vi "Get extended drive and motor status.vi"(0 "COM port":refnum<visa-resource-name>, 1 "Drive address":T5=1 items=["0", "1", "2", "3", "4", "5", "6", "7", "8", "9", "10", "11", "12", "13", "14", "15", "16", "17", "18", "19", "20", "21", "22", "23", "24", "25", "26", "27", "28", "29", "30", "31", "32", "33", "34", "35", "36", "37", "38", "39", "40", "41", "42", "43", "44", "45", "46", "47", "48", "49", "50", "51", "52", "53", "54", "55", "56", "57", "58", "59", "60", "61", "62", "63"]) -> (3 "No errors":bool, 4 "Modbus error cluster":T1={"Checksum ok"=FALSE, "Modbus exception code"=1, "Response from correct drive"=FALSE, "Comms error"={"status"=FALSE, "code"=0, "source"=""}} {"Modbus exception code" items=["None"=0, "Invalid function request"=1, "Invalid Modbus register address"=2, "Invalid / unauthorised data value"=3, "Device failure"=4, "Request accepted, wait"=5, "Drive busy"=6, "Request rejected"=7, "Memory parity error"=8, "Gateway path unavailable"=10, "Device failed to respond"=11]}, 5 "Extended drive status":T4, 6 "Motor data":T3)   [LabVIEW 2020]
doc: "Modbus RTU for Invertek drives. Paul Nathan 21-JUN-2022."
uses:
  ctls/Drive address.ctl
  ctls/Extended drive status bits.ctl
  ctls/Motor data.ctl
  ctls/Modbus error cluster.ctl
  ctls/Exception codes.ctl
  ctls/Register.ctl
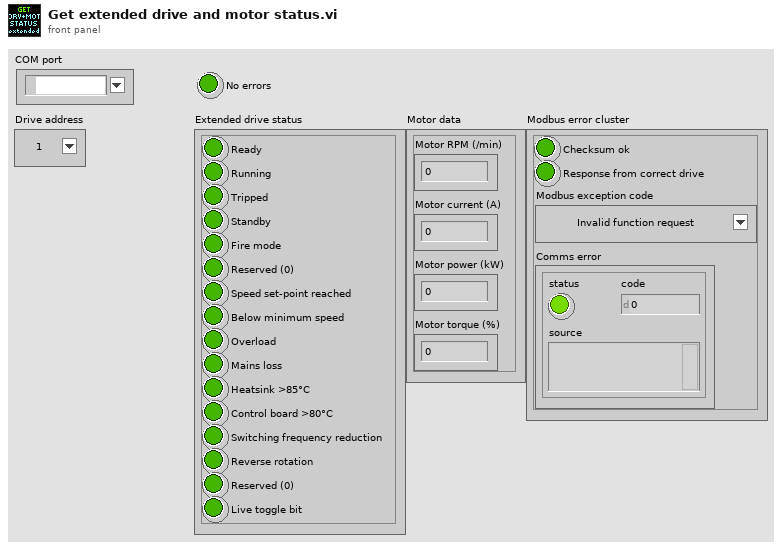
[diagram p1: front panel]
types:
  T1 = typedef "Modbus error cluster.ctl" = cluster{"Checksum ok":bool, "Modbus exception code":T2, "Response from correct drive":bool, "Comms error":errorcluster}
  T2 = typedef "Exception codes.ctl" = u8
  T3 = typedef "Motor data.ctl" = cluster{"Motor RPM (/min)":dbl, "Motor current (A)":dbl, "Motor power (kW)":dbl, "Motor torque (%)":dbl}
  T4 = typedef "Extended drive status bits.ctl" = cluster{"Ready":bool, "Running":bool, "Tripped":bool, "Standby":bool, "Fire mode":bool, "Reserved (0)":bool, "Speed set-point reached":bool, "Below minimum speed":bool, "Overload":bool, "Mains loss":bool, "Heatsink >85°C":bool, "Control board >80°C":bool, "Switching frequency reduction":bool, "Reverse rotation":bool, "Reserved (0)":bool, "Live toggle bit":bool}
  T5 = typedef "Drive address.ctl" = u8
  T6 = typedef "Register.ctl" = u16
  T7 = cluster{"Boolean array[0]":bool, "Boolean array[1]":bool, "Boolean array[2]":bool, "Boolean array[3]":bool, "Boolean array[4]":bool, "Boolean array[5]":bool, "Boolean array[6]":bool, "Boolean array[7]":bool, "Boolean array[8]":bool, "Boolean array[9]":bool, "Boolean array[10]":bool, "Boolean array[11]":bool, "Boolean array[12]":bool, "Boolean array[13]":bool, "Boolean array[14]":bool, "Boolean array[15]":bool}
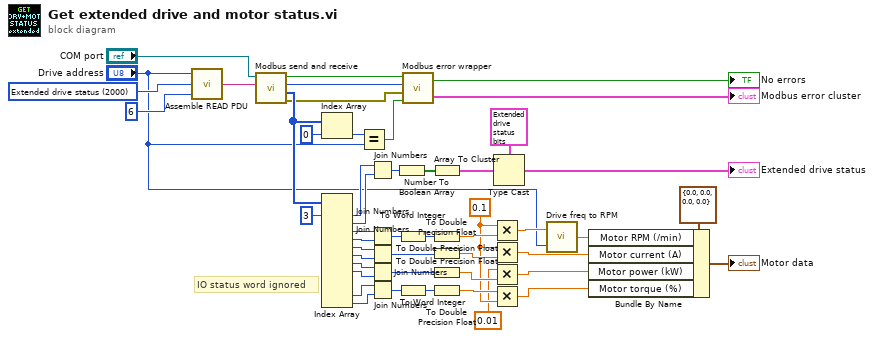
[diagram p0: block diagram]
diagram:
  w11 = T6 2000 items=["Control"=0, "RPM set-point"=4, "Drive status"=5, "Output RPM"=6, "Motor current"=7, "Motor torque"=8, "Motor power"=9, "DC bus voltage"=22, "Drive power stage temperature"=23, "kWh meter"=31, "MWh meter"=32, "Running time - hours"=33, "Running time - seconds"=34, "Internal drive temperature"=38, "Motor RMS voltage"=42, "Extended drive status"=2000] ("Register")
  w13 = 0.1 ("y")
  # "IO status word ignored"
  n1 = call "Assemble READ PDU.vi"("No. of registers"=u16 6, "Register"=w11, "Drive address"="Drive address") -> ("Ser out string"=w49:string)
  n2 = call "Modbus send and receive.vi"("Modbus telegram"=w49, "COM port"="COM port") -> ("Comms error"=w2:errorcluster, "Device response"=w44:u8[], "Modbus exception code"=w3:T2, "Checksum ok"=w4:bool)  [unwired: 2 in]
  n3 = Index Array(array=w44, index=0) -> (element=w46:u8)
  n4 = Index Array(array=w44, index #1=3 ("index")) -> (element #1=w38:u8, element #2=w37:u8, element #3=w24:u8, element #4=w23:u8, element #5=w22:u8, element #6=w21:u8, element #7=w20:u8, element #8=w19:u8, element #11=w18:u8, element #12=w17:u8)  [unwired: 11 in, 2 out]
  n5 = Equal?(x=w46, y="Drive address") -> (x = y?=w1:bool)
  n6 = Join Numbers(hi=w38, lo=w37) -> ((hi.lo)=w36:u16)
  n7 = Join Numbers(hi=w24, lo=w23) -> ((hi.lo)=w25:u16)
  n8 = Join Numbers(hi=w22, lo=w21) -> ((hi.lo)=w28:u16)
  n9 = Join Numbers(hi=w20, lo=w19) -> ((hi.lo)=w14:u16)
  n10 = Join Numbers(hi=w18, lo=w17) -> ((hi.lo)=w16:u16)
  n11 = Number To Boolean Array(number=w36) -> (Boolean array=w42:bool[])
  n12 = To Word Integer(number=w25) -> (16bit integer=w26:i16)
  n13 = To Word Integer(number=w16) -> (16bit integer=w15:i16)
  n14 = call "Modbus error wrapper.vi"("Response from correct drive"=w1, "Comms error"=w2, "Modbus exception code"=w3, "Checksum ok"=w4) -> ("Modbus error cluster"=→"Modbus error cluster":T1, "No errors"=→"No errors":bool)
  n15 = Array To Cluster(array=w42) -> (cluster=w41:T7)
  n16 = To Double Precision Float(number=w26) -> (double precision float=w29:dbl)
  n17 = To Double Precision Float(number=w28) -> (double precision float=w30:dbl)
  n18 = To Double Precision Float(number=w14) -> (double precision float=w31:dbl)
  n19 = To Double Precision Float(number=w15) -> (double precision float=w32:dbl)
  n20 = Multiply(x=w13, y=w29) -> (x*y=w10:dbl)
  n21 = Multiply(x=w13, y=w30) -> (x*y=w33:dbl)
  n22 = Multiply(x=0.01 ("y"), y=w31) -> (x*y=w34:dbl)
  n23 = Multiply(x=w32, y=w13) -> (x*y=w35:dbl)
  n24 = Type Cast(type=T4 {"Ready"=FALSE, "Running"=FALSE, "Tripped"=FALSE, "Standby"=FALSE, "Fire mode"=FALSE, "Reserved (0)"=FALSE, "Speed set-point reached"=FALSE, "Below minimum speed"=FALSE, "Overload"=FALSE, "Mains loss"=FALSE, "Heatsink >85°C"=FALSE, "Control board >80°C"=FALSE, "Switching frequency reduction"=FALSE, "Reverse rotation"=FALSE, "Reserved (0)"=FALSE, "Live toggle bit"=FALSE} ("Extended drive status bits"), x=w41) -> (*(type *) &x=→"Extended drive status":T4)
  n25 = call "Drive freq to RPM.vi"("Drive address"="Drive address", "Drive output f (Hz)"=w10) -> ("Motor RPM (/min)"=w9:dbl)
  n26 = Bundle By Name(cluster=T3 {"Motor RPM (/min)"=0.0, "Motor current (A)"=0.0, "Motor power (kW)"=0.0, "Motor torque (%)"=0.0} ("Motor stats"), "Motor RPM (/min)"=w9, "Motor current (A)"=w33, "Motor power (kW)"=w34, "Motor torque (%)"=w35) -> (→"Motor data":T3)
